vi "操作Sql的Sample-simple.vi"(3 "SavefileName":string="C:\\0000.txt", 6 "sn 2":string="SFP+ 002", 7 "fieldName":string="S4P10G", 8 "下载文件":bool, 9 "fileName":string="C:\\9999.txt", 10 "fieldName_Index":string="S4P10G", 11 "sn":string="SFP+ 002") -> ()   [LabVIEW 2011]
uses:
  ClassLibrary_Sql 1.2.dll
panel:
  out "UpdateStreamFileToSql":bool
  out "StreamFileToSql":bool
  in  "fieldName_Sn 2":string="FixtureNo"
  in  "fieldName_Sn":string="FixtureNo"
  in  "tableName":string="vfixture"
  out "GetFileFromSql":bool
  out "SelectTheRecordIsExist 2":bool
  out "SelectTheRecordIsExist":bool
  # "查询和上传文件"
  # "查询和下载文件"
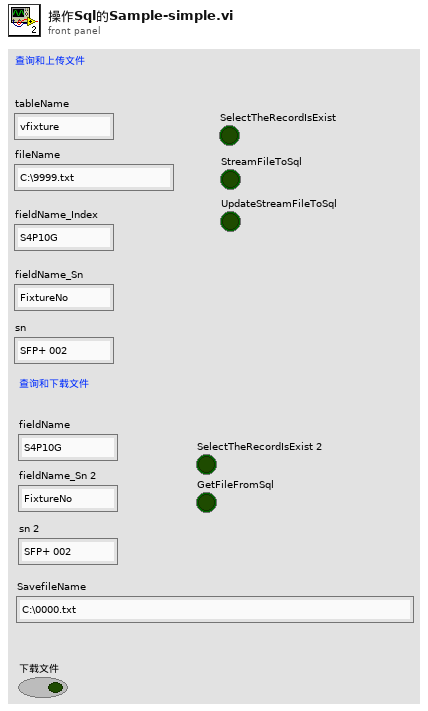
[diagram p1: front panel]
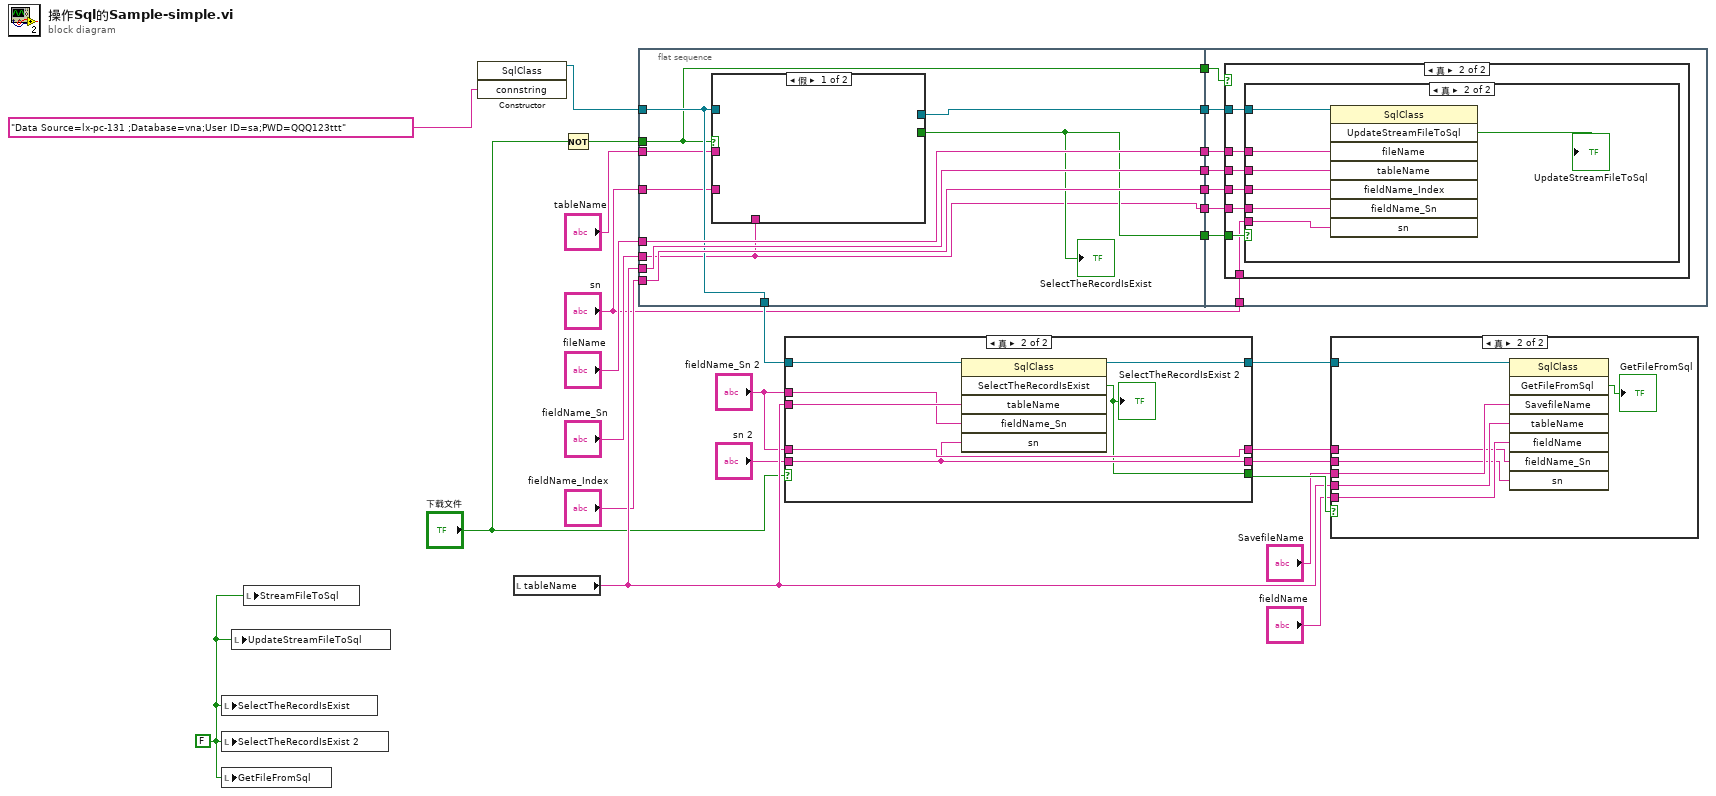
[diagram p0: block diagram]
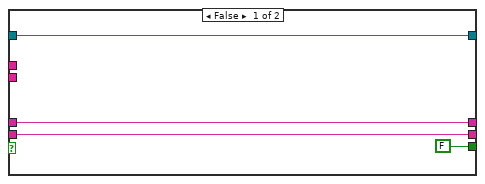
[diagram p3: hidden frame]
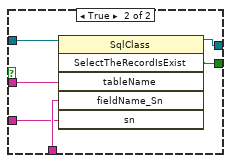
[diagram p4: hidden frame]
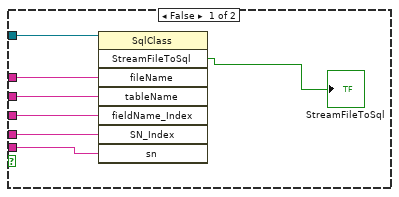
[diagram p6: hidden frame]
diagram:
  w6 = FALSE
  n1 = local write "SelectTheRecordIsExist"(w6) -> ()
  n2 = local write "SelectTheRecordIsExist 2"(w6) -> ()
  n3 = local write "GetFileFromSql"(w6) -> ()
  n4 = local write "UpdateStreamFileToSql"(w6) -> ()
  n5 = local write "StreamFileToSql"(w6) -> ()
  n6 = constructor class="SqlClass"("connstring"="Data Source=lx-pc-131 ;Database=vna;User ID=sa;PWD=QQQ123ttt") -> (reference out=w4:refnum<k24>)  [unwired: 3 in, 3 out]
  n7 = local read "tableName"() -> (w21:string)
  n8 = Not(x="下载文件") -> (.not. x?=w3:bool)
  n9 = flat-sequence {
    tunnel: [w32] -> w27
    tunnel: [w34] -> w26
    tunnel: "tableName" -> [w31]
    tunnel: w21 -> [w36]
    tunnel: [w36] -> w22
    tunnel: "fileName" -> [w35]
    tunnel: [w35] -> w19
    tunnel: "fieldName_Index" -> [w37]
    tunnel: [w37] -> w17
    tunnel: "fieldName_Sn" -> [w30]
    tunnel: [w30] -> w15
    tunnel: "sn" -> [w29]
    tunnel: [w33] -> w8
    tunnel: w4 -> [w34]
    tunnel: w3 -> [w28]
    tunnel: [w28] -> w1
    tunnel: w27 -> [w51]
    tunnel: w22 -> [w50]
    tunnel: w19 -> [w49]
    tunnel: w17 -> [w48]
    tunnel: w15 -> [w47]
    tunnel: "sn" -> [w46]
    tunnel: w8 -> [w45]
    tunnel: w1 -> [w44]
    frame #0 {
      n10 = case shown="假" w28 {
        tunnel: w34 -> [_ w43]
        tunnel: [_ w42] -> w33
        tunnel: [_ w41] -> w32
        tunnel: w31 -> [_ w40]
        tunnel: w30 -> [_ w39]
        tunnel: w29 -> [_ w38]
        frame False {
        }
        frame True {
          n11 = invoke class="SqlClass" method="SelectTheRecordIsExist"(reference=w43, "tableName"=w40, "fieldName_Sn"=w39, "sn"=w38) -> (reference out=w42:refnum<k24>, "SelectTheRecordIsExist"=w41:bool)  [unwired: 2 in, 4 out]
        }
      }
      "SelectTheRecordIsExist" <- w32
    }
    frame #1 {
      n12 = case shown="真" w44 {
        tunnel: w51 -> [_ w58]
        tunnel: w50 -> [_ w57]
        tunnel: w49 -> [_ w56]
        tunnel: w48 -> [_ w55]
        tunnel: w47 -> [_ w54]
        tunnel: w46 -> [_ w53]
        tunnel: w45 -> [_ w52]
        frame False {
        }
        frame True {
          n13 = case shown="真" w58 {
            tunnel: w57 -> [w63 w70]
            tunnel: w56 -> [w64 w71]
            tunnel: w55 -> [w61 w69]
            tunnel: w54 -> [w60 w68]
            tunnel: w53 -> [w62 w67]
            tunnel: w52 -> [w65 w72]
            frame False {
              n14 = invoke class="SqlClass" method="StreamFileToSql"(reference=w65, "fileName"=w64, "tableName"=w63, "fieldName_Index"=w61, "SN_Index"=w60, "sn"=w62) -> ("StreamFileToSql"=→"StreamFileToSql":bool)  [unwired: 2 in, 7 out]
            }
            frame True {
              n15 = invoke class="SqlClass" method="UpdateStreamFileToSql"(reference=w72, "fileName"=w71, "tableName"=w70, "fieldName_Index"=w69, "fieldName_Sn"=w68, "sn"=w67) -> ("UpdateStreamFileToSql"=→"UpdateStreamFileToSql":bool)  [unwired: 2 in, 7 out]
            }
          }
        }
      }
    }
  }
  n16 = case shown="真" "下载文件" {
    tunnel: w26 -> [w75 w82]
    tunnel: [FALSE ("SelectTheRecordIsExist") w78] -> w25
    tunnel: [w75 w77] -> w24
    tunnel: w21 -> [_ w81]
    tunnel: "fieldName_Sn 2" -> [_ w80]
    tunnel: "sn 2" -> [w74 w79]
    tunnel: [w76 w83] -> w13
    tunnel: "fieldName_Sn 2" -> [w76 w83]
    tunnel: [w74 w79] -> w11
    frame False {
    }
    frame True {
      n17 = invoke class="SqlClass" method="SelectTheRecordIsExist"(reference=w82, "tableName"=w81, "fieldName_Sn"=w80, "sn"=w79) -> (reference out=w77:refnum<k24>, "SelectTheRecordIsExist"=w78:bool)  [unwired: 2 in, 4 out]
      "SelectTheRecordIsExist 2" <- w78
    }
  }
  n18 = case shown="真" w25 {
    tunnel: w24 -> [_ w90]
    tunnel: w21 -> [_ w88]
    tunnel: w13 -> [_ w86]
    tunnel: "fieldName" -> [_ w87]
    tunnel: w11 -> [_ w85]
    tunnel: "SavefileName" -> [_ w89]
    frame False {
    }
    frame True {
      n19 = invoke class="SqlClass" method="GetFileFromSql"(reference=w90, "SavefileName"=w89, "tableName"=w88, "fieldName"=w87, "fieldName_Sn"=w86, "sn"=w85) -> ("GetFileFromSql"=→"GetFileFromSql":bool)  [unwired: 2 in, 7 out]
    }
  }
